vi "VariableWrite.vi"(8 "error in (no error)":errorcluster, 9 "OriginalName":string, 10 "Variable":refnum<class "Variable.lvclass">, 11 "VariableManagerRef in":refnum<vi>) -> (0 "error out":errorcluster, 3 "VariableManagerRef out":refnum<vi>)   [LabVIEW 2013, in "VariableManagerAPI.lvlib"]
doc: "Add the given variable definition to database.\nTo overwrite existing variable definition, provide the OriginalName.\n\nAn error is thrown if the given Variable is malformed, failing the test in VariableCheck.vi"
uses:
  VariableManagerAPI.lvlib
  VariableManager/VariableManager.lvclass
  Variable/Variable.lvclass
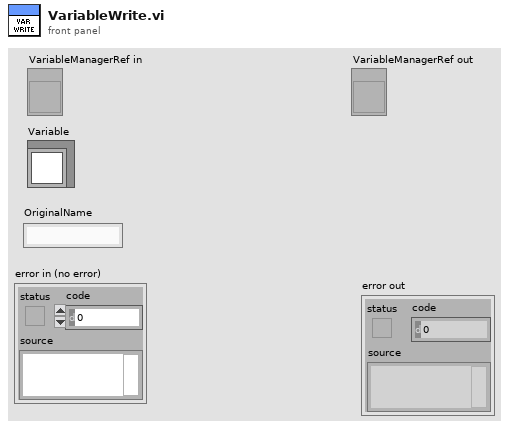
[diagram p1: front panel]
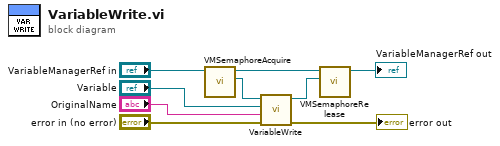
[diagram p0: block diagram]
diagram:
  n1 = call "VMSemaphoreAcquire.vi"("VariableManagerRef in"="VariableManagerRef in") -> ("VariableManager"=w9:refnum<class "VariableManager.lvclass">, "VariableManagerRef out"=w7:refnum<vi>)  [unwired: 7 in, 2 out]
  n2 = call-dynamic "VariableWrite.vi"("error in (no error)"="error in (no error)", "OriginalName"="OriginalName", "Variable"="Variable", "VariablesManager in"=w9) -> ("error out"=→"error out":errorcluster, "VariablesManager out"=w3:refnum<class "VariableManager.lvclass">)  [unwired: 6 in]
  n3 = call "VMSemaphoreRelease.vi"("VariableManager"=w3, "VariableManagerRef in"=w7) -> ("VariableManagerRef out"=→"VariableManagerRef out":refnum<vi>)  [unwired: 8 in, 1 out]
